vi "Test_Second_max.vi"() -> ()   [LabVIEW 2022 SP3]
panel:
  out "AP3":dbl
  in  "Array":dbl[](array[numeric])
  in  "stop":bool
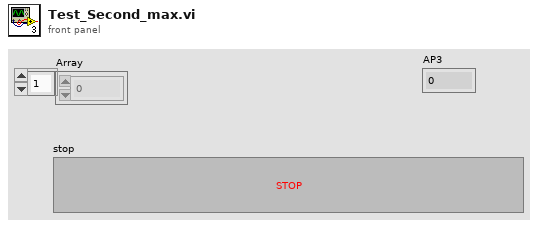
[diagram p1: front panel]
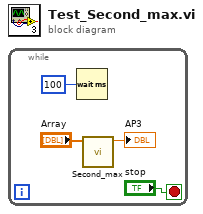
[diagram p0: block diagram]
diagram:
  n1 = while {
    stop <- "stop" stop-if-true
    n2 = Wait (ms)(milliseconds to wait=u32 100) -> ()  [unwired: 1 out]
    n3 = call "Second_max.vi"("Array"="Array") -> ("AP3"=→"AP3":dbl)  [unwired: 10 in]
  }
